vi "UpdateInspect.vi"(6 "Current Id":i32, 8 "Answers":T1, 9 "Current Z":dbl, 10 "Displacements":dbl[](array[numeric]), 11 "Inspect? in":bool[](array[boolean])) -> (3 "Inspect? out":bool[](array[boolean]))   [LabVIEW 2014]
panel:
  out "?":cluster{i32[], dbl[]}[](graph)
  # "LICENSED MATERIALS – PROPERTY OF IBM\nCopyright IBM Corp. 2016,\nALL RIGHTS RESERVED"
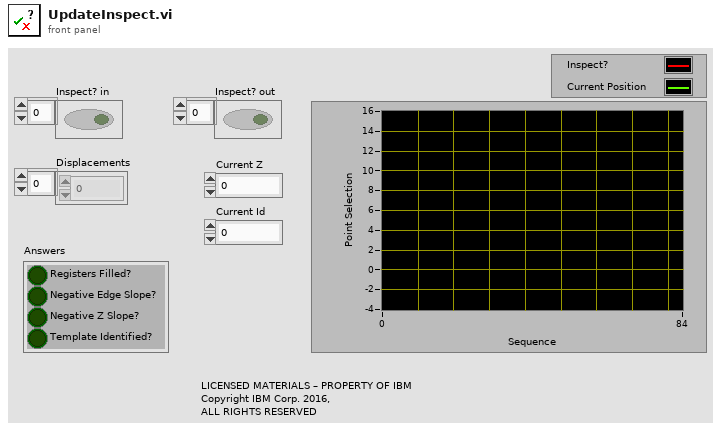
[diagram p1: front panel]
types:
  T1 = cluster{"Registers Filled?":bool, "Negative Edge Slope?":bool, "Negative Z Slope?":bool, "Template Identified?":bool}
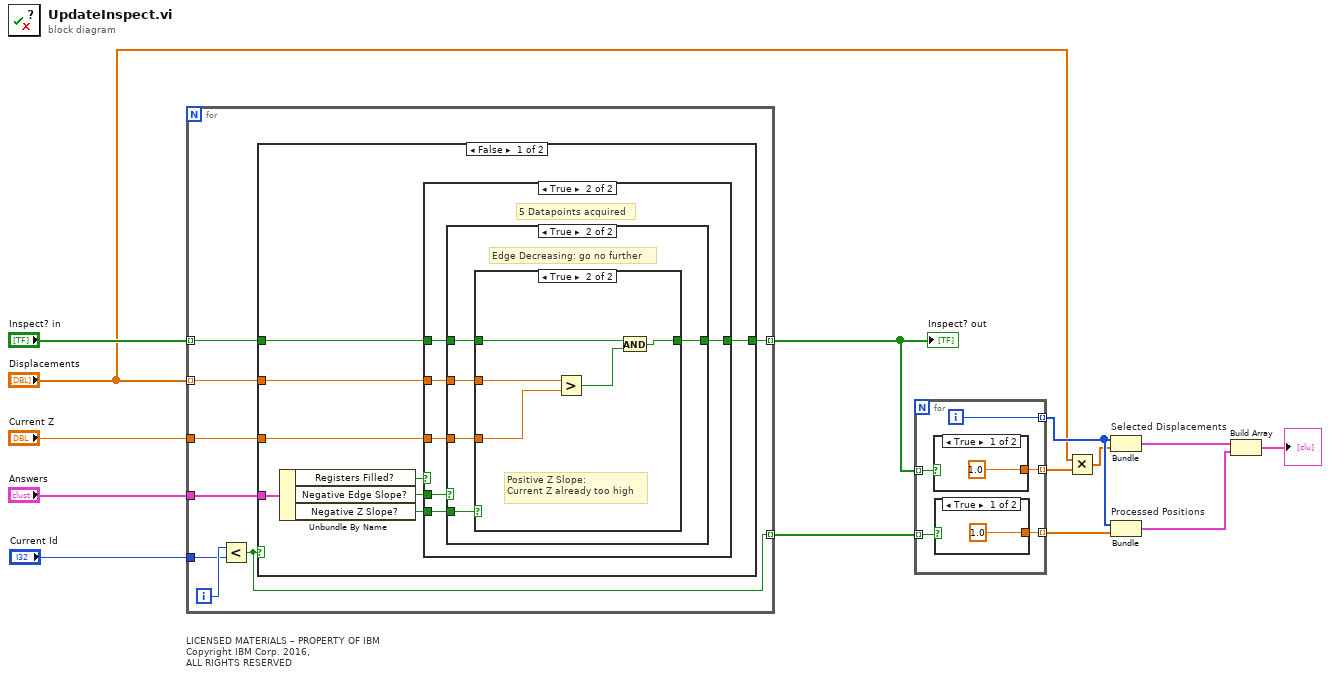
[diagram p0: block diagram]
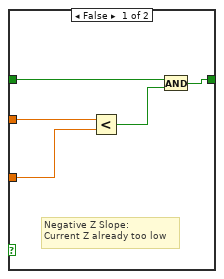
[diagram p4: hidden frame]
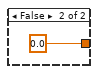
[diagram p6: hidden frame]
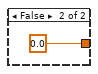
[diagram p7: hidden frame]
diagram:
  # "LICENSED MATERIALS – PROPERTY OF IBM\nCopyright IBM Corp. 2016,\nALL RIGHTS RESERVED"
  n1 = for {
    tunnel: "Displacements" -> [w22] mode=indexing
    tunnel: "Answers" -> [w21]
    tunnel: "Inspect? in" -> [w20] mode=indexing
    tunnel: "Current Z" -> [w19]
    tunnel: [w18] -> w11 mode=indexing
    tunnel: "Current Id" -> [w16]
    tunnel: [w15] -> w8 mode=indexing
    i -> [w17]
    n2 = Less?(x=w17, y=w16) -> (x < y?=w15:bool)
    n3 = case shown="False" w15 {
      tunnel: w22 -> [w30 _]
      tunnel: w21 -> [w28 _]
      tunnel: w20 -> [w27 w54]
      tunnel: w19 -> [w24 _]
      tunnel: [w23 w54] -> w18
      frame False {
        n4 = Unbundle By Name(w28) -> ("Registers Filled?"=w29:bool, "Negative Edge Slope?"=w26:bool, "Negative Z Slope?"=w25:bool)
        n5 = case shown="True" w29 {
          tunnel: w27 -> [w31 w35]
          tunnel: [w31 w34] -> w23
          tunnel: w30 -> [_ w33]
          tunnel: w26 -> [_ w37]
          tunnel: w25 -> [_ w36]
          tunnel: w24 -> [_ w32]
          frame False {
            # "Wait for until 5 datapoints are aquired"
          }
          frame True {
            # "5 Datapoints acquired"
            n6 = case shown="True" w37 {
              tunnel: w36 -> [_ w43]
              tunnel: w35 -> [w38 w42]
              tunnel: [w38 w41] -> w34
              tunnel: w33 -> [_ w40]
              tunnel: w32 -> [_ w39]
              frame False {
                # "Edge Increasing: Keep marching"
              }
              frame True {
                # "Edge Decreasing: go no further"
                n7 = case shown="True" w43 {
                  tunnel: w42 -> [w48 w53]
                  tunnel: [w47 w52] -> w41
                  tunnel: w40 -> [w46 w51]
                  tunnel: w39 -> [w45 w50]
                  frame False {
                    # "Negative Z Slope:\nCurrent Z already too low"
                    n8 = Less?(x=w46, y=w45) -> (x < y?=w44:bool)
                    n9 = And(x=w48, y=w44) -> (x .and. y?=w47:bool)
                  }
                  frame True {
                    # "Positive Z Slope:\nCurrent Z already too high"
                    n10 = Greater?(x=w51, y=w50) -> (0:w49:bool)
                    n11 = And(x=w53, y=w49) -> (x .and. y?=w52:bool)
                  }
                }
              }
            }
          }
        }
      }
      frame True {
      }
    }
  }
  "Inspect? out" <- w11
  n12 = for {
    tunnel: w11 -> [w59] mode=indexing
    tunnel: [w58] -> w3 mode=indexing
    tunnel: [w57] -> w6 mode=indexing
    tunnel: w8 -> [w56] mode=indexing
    tunnel: [w55] -> w7 mode=indexing
    i -> [w57]
    n13 = case shown="True" w59 {
      tunnel: [1.0 0.0] -> w58
      frame True {
      }
      frame False {
      }
    }
    n14 = case shown="True" w56 {
      tunnel: [1.0 0.0] -> w55
      frame True {
      }
      frame False {
      }
    }
  }
  n15 = Multiply(x="Displacements", y=w3) -> (x*y=w1:dbl[])
  n16 = Bundle "Selected Displacements"(w6, w1) -> (w10:cluster{i32[], dbl[]})  [unwired: 1 in]
  n17 = Bundle "Processed Positions"(w6, w7) -> (w4:cluster{i32[], dbl[]})  [unwired: 1 in]
  n18 = Build Array(w10, w4) -> (→"?":cluster{i32[], dbl[]}[])
